vi "microfluidic_paper_controller_V1.vi"() -> ()   [LabVIEW 2016]
uses:
  <userlib>/Fluigent/Fluigent MFCS/FluigentMFCS_Full.llb/MFCS_EZ Detect.vi
  <userlib>/Fluigent/Fluigent MFCS/FluigentMFCS_Full.llb/MFCS_EZ Initialization.vi
  Gss.vi
  <vilib>/imath/engines/lvmath2/RunTimeEngine/ArithmeticOperatorToken/NIMS_ArithmeticOperator_multmx(M,CV).vi
  <instcachedir>/0/NIMS_ArithmeticOperator_multmx(M,CV)_4D43781A51B54AFABA7ECA2AD711762F.lvgen/NIMS_ArithmeticOperator_multmx(M,CV)_4D43781A51B54AFABA7ECA2AD711762F_000.vi
  <vilib>/imathl/engines/lvmath/Functions/Error Handling/Create Error.vi
  <vilib>/imath/engines/lvmath2/RunTimeEngine/IndexRead/NIMS M(R2).vi
  <instcachedir>/0/NIMS M(R2)_287818D58BD74005B29FE73CE7602B1A.lvgen/NIMS M(R2)_287818D58BD74005B29FE73CE7602B1A_000.vi
  <vilib>/imath/engines/lvmath2/RunTimeEngine/NodeEndStatement/NIMS_NodeEndStatement_Get Vector.vi
  <instcachedir>/0/NIMS_NodeEndStatement_Get Vector_6D35898B950C4E42AD3C631ACA708625.lvgen/NIMS_NodeEndStatement_Get Vector_6D35898B950C4E42AD3C631ACA708625_001.vi
  <vilib>/imath/engines/lvmath2/RunTimeEngine/NodeEndStatement/NIMS_NodeEndStatement_Output.vi
  <instcachedir>/0/NIMS_NodeEndStatement_Output_53EC0D466D134D7ABD903AC30B43404B.lvgen/NIMS_NodeEndStatement_Output_53EC0D466D134D7ABD903AC30B43404B_005.vi
  <vilib>/imath/engines/lvmath2/RunTimeEngine/ErrorHandling/NIMS_Finalize Error.vi
  <userlib>/Fluigent/Fluigent MFCS/FluigentMFCS_Full.llb/MFCS_EZ Read All Channels Pressure.vi
  <userlib>/Fluigent/Fluigent MFCS/FluigentMFCS_Full.llb/MFCS_EZ Write Channel Pressure.vi
  <userlib>/Fluigent/Fluigent MFCS/FluigentMFCS_Full.llb/MFCS_EZ Close.vi
  <vilib>/Analysis/NI_AALBase.lvlib
  <vilib>/Analysis/baseanly.llb/Mean (DBL).vi
panel:
  in  "alpha":dbl
  in  "milliseconds to wait":u32=50
  out "Set Pressure":dbl[](array[numeric])=[400.0, 400.0]
  out "Flow 1 plot 2":cluster{"[0]":dbl, "[1]":dbl}(graph)={"[0]"=400.0, "[1]"=636.4874575000703}
  out "Flow Rates":dbl[](array[numeric])=[1099.9989421021717, 636.4874575000703]
  in  "Ftot Setpoint":dbl=400.0
  in  "Vals to display":dbl=1235.0
  out "Flow 1 plot":cluster{"[0]":dbl, "[1]":dbl}(graph)={"[0]"=1099.9989421021717, "[1]"=300.0}
  out "Ferr":T1(graph)={"output[0]"=-2.2986299232843663, "output[1]"=-0.9866301071552578, "output[2]"=0.0}
  out "Pressures":dbl[](array[numeric])=[404.58697509765625, 396.3816223144531]
  in  "reset Averging":bool
  in  "Set current Pressure\n to manual pressure":bool
  out "Pressures":T2(graph)={"[0]"=404.58697509765625, "[1]"=396.3816223144531, "[2]"=400.0, "[3]"=400.0}
  in  "stop":bool=TRUE
  in  "Control Valves":enum16{"1", "2", "3", "4", "5", "6", "7", "8"}[](array[ring])=[enum."7", enum."8"]
  in  "Pressure Channels":i16[](array[numeric])=[2, 3]
  in  "Manual Pressure Set":dbl[](array[numeric])=[400.0, 400.0]
  in  "Control On":bool
  in  "F1 Setpoint":dbl=300.0
  in  "Add Ctrl?":bool
  in  "Boards":enum16{"A", "B", "C"}[](array[ring])=[enum."A", enum."A"]
  in  "Valves":enum16{"1", "2", "3", "4", "5", "6", "7", "8"}[](array[ring])=[enum."5", enum."1"]
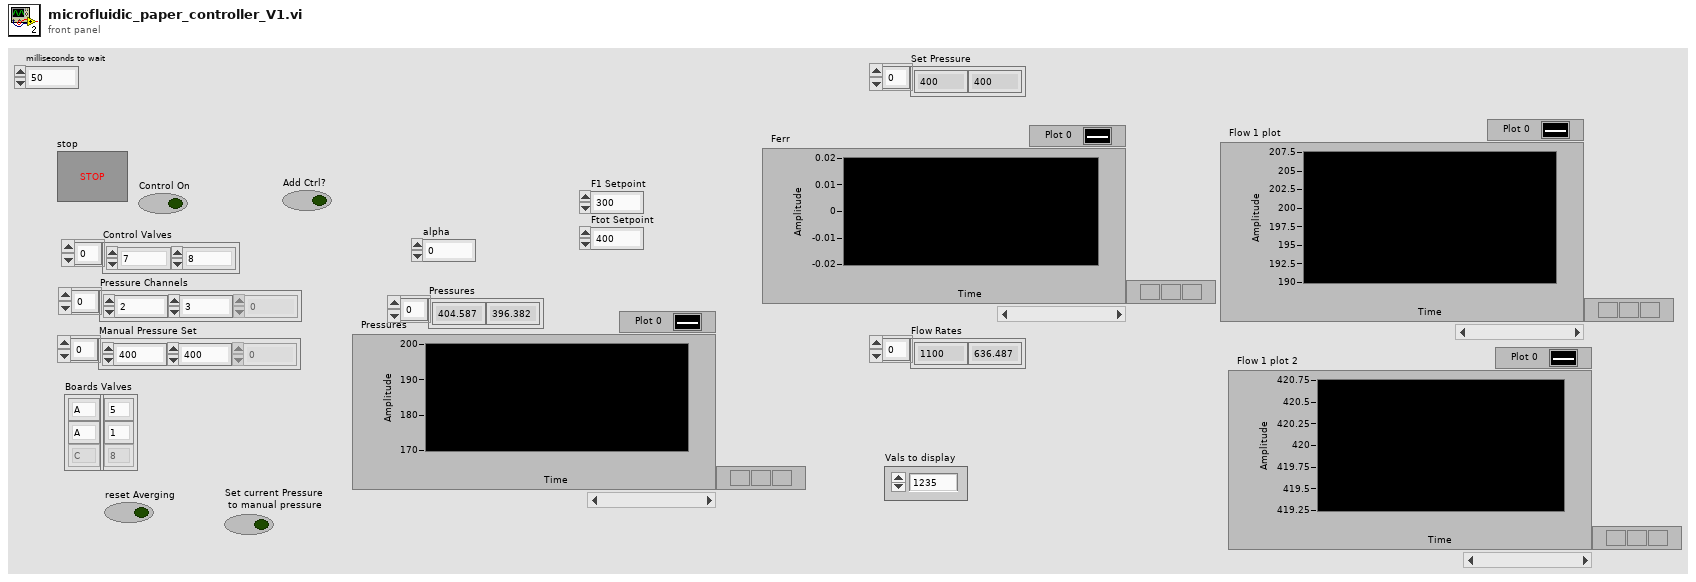
[diagram p1: front panel]
types:
  T1 = cluster{"output[0]":dbl, "output[1]":dbl, "output[2]":dbl}
  T2 = cluster{"[0]":dbl, "[1]":dbl, "[2]":dbl, "[3]":dbl}
  T3 = cluster{"relative seconds":dbl, "Pressures":dbl[], "F1 PID gains":dbl[], "FTot PID gains":dbl[], "PID On?":i16}
  T4 = typedef "_EZmfcsSN.ctl" = u16
  T5 = typedef "_EZmfcsRefNum.ctl" = refnum<k1>
  T6 = cluster{"setpoint high":dbl, "setpoint low":dbl}[]
  T7 = cluster{"err[0]":dbl, "err[1]":dbl, "err[2]":dbl}
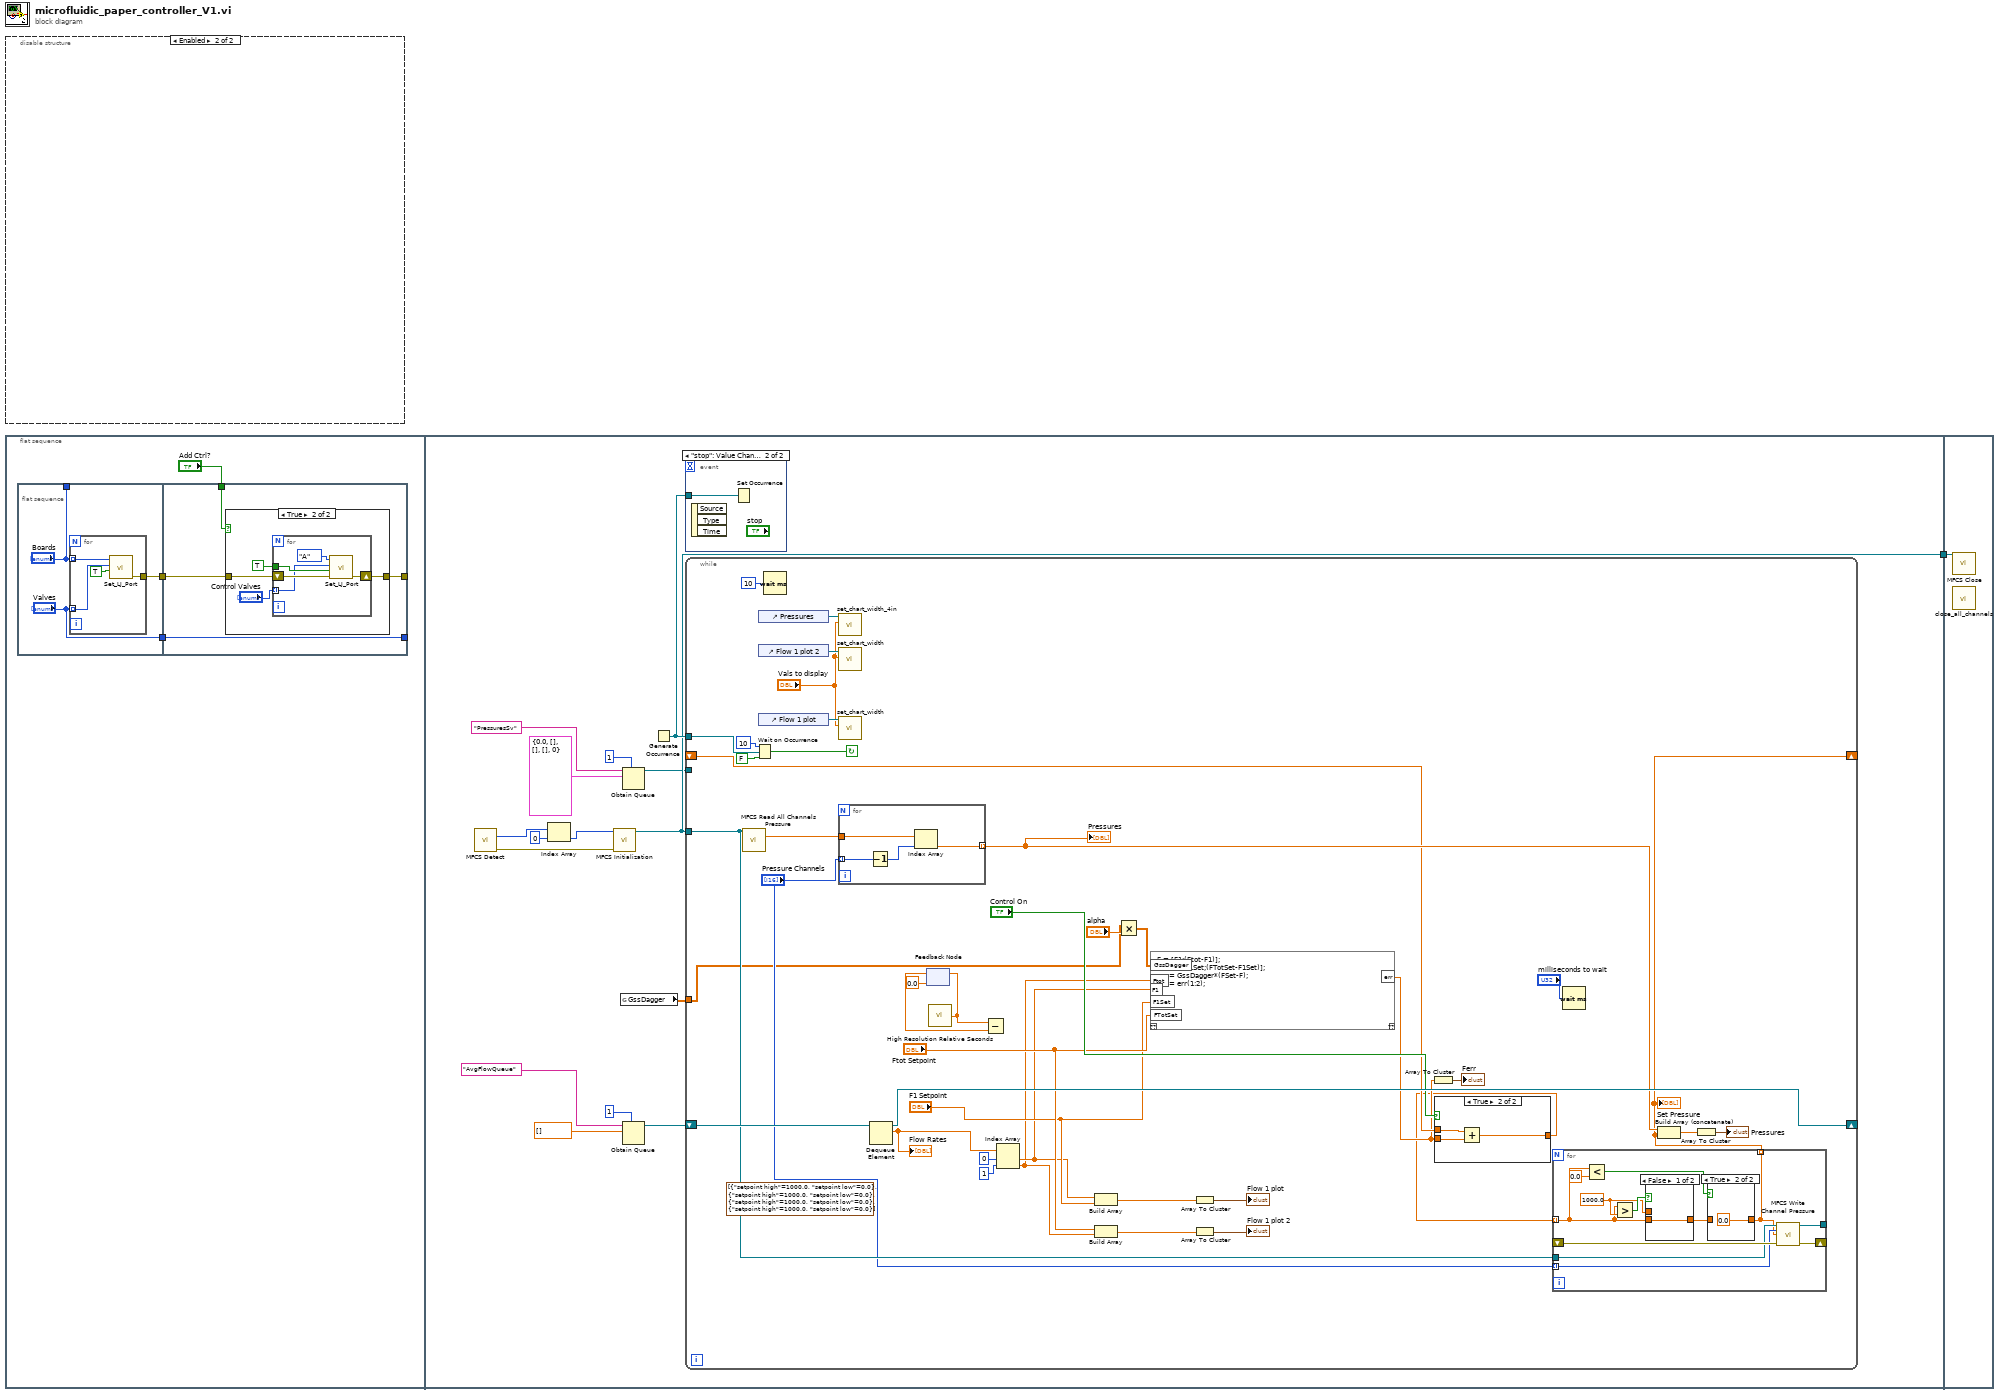
[diagram p0: block diagram]
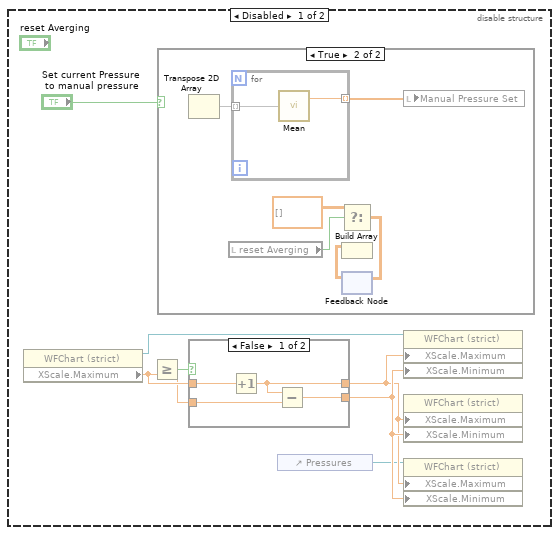
[diagram p2: hidden frame]
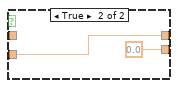
[diagram p3: hidden frame]
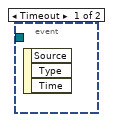
[diagram p6: hidden frame]
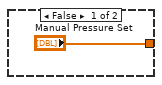
[diagram p9: hidden frame]
diagram:
  n1 = disable-structure shown="Enabled" {
    frame Disabled {
      n2 = property on="Property Node" class="WFChart (strict)"() -> (reference=w5:refnum<vi>, reference out=w6:refnum<vi>, "XScale.Maximum"=w4:dbl)  [unwired: 1 in, 1 out]
      n3 = Greater Or Equal?(y=w4) -> (x=w2:dbl, x >= y?=w3:bool)
      n4 = case shown="True" "Set current Pressure\n to manual pressure" {
        frame False {
        }
        frame True {
          n5 = Transpose 2D Array() -> (transposed array=w21:dbl[][])  [unwired: 1 in]
          n6 = local read "reset Averging"() -> (w22:bool)
          n7 = for {
            tunnel: w21 -> [w25] mode=indexing
            tunnel: [w24] -> w18 mode=indexing
            n8 = call-poly <vilib>:"Mean.vi"("X"=w25) -> ("mean"=w24:dbl)  [unwired: 1 out]
          }
          n9 = Select(t=dbl[][] [] ("appended array"), s=w22) -> (s? t:f=w19:dbl[][])  [unwired: 1 in]
          n10 = feedback-in #1(w19) -> ()
          n11 = feedback #1() -> (w23:dbl[][])  [unwired: 1 in]
          n12 = Build Array(w23) -> ()  [unwired: 1 in, 1 out]
          n13 = local write "Manual Pressure Set"(w18) -> ()
        }
      }
      n14 = case shown="False" w3 {
        tunnel: w2 -> [w13 w17]
        tunnel: w4 -> [w15 _]
        tunnel: [w12 w17] -> w9
        tunnel: [w14 0.0] -> w10
        frame False {
          n15 = Increment(x=w15) -> (x+1=w12:dbl)
          n16 = Subtract(x=w12, y=w13) -> (x-y=w14:dbl)
        }
        frame True {
        }
      }
      n17 = control-ref of="Pressures"() -> (w7:refnum<vi>)
      n18 = property on="Property Node" class="WFChart (strict)"(reference=w6, "XScale.Maximum"=w9, "XScale.Minimum"=w10) -> ()  [unwired: 1 in, 2 out]
      n19 = property on="Property Node" class="WFChart (strict)"("XScale.Maximum"=w9, "XScale.Minimum"=w10) -> (reference=w8:refnum<vi>)  [unwired: 1 in, 2 out]
      n20 = property on="Property Node" class="WFChart (strict)"(reference=w7, "XScale.Maximum"=w9, "XScale.Minimum"=w10) -> ()  [unwired: 1 in, 2 out]
    }
    frame Enabled {
    }
  }
  n21 = flat-sequence {
    tunnel: [w55] -> w1
    tunnel: w1 -> [w212]
    frame #0 {
      n22 = flat-sequence {
        tunnel: ["Boards"] -> _
        tunnel: [w31] -> w28
        tunnel: ["Valves"] -> w27
        tunnel: [w39] -> _
        tunnel: [w37] -> _
        tunnel: w28 -> [w38]
        tunnel: w27 -> [w39]
        tunnel: "Add Ctrl?" -> [w36]
        frame #0 {
          n23 = for {
            tunnel: "Valves" -> [w35] mode=indexing
            tunnel: "Boards" -> [w34] mode=indexing
            tunnel: [w32] -> w31
            n24 = call "Set_LJ_Port.vi"("State"=TRUE, "Channel"=w35, "Flowboard"=w34) -> ("error out"=w32:errorcluster)  [unwired: 8 in]
          }
        }
        frame #1 {
          n25 = case shown="True" w36 {
            tunnel: w38 -> [w40 w44]
            tunnel: [w40 w43] -> w37
            frame False {
            }
            frame True {
              n26 = for {
                tunnel: TRUE ("State") -> [w47]
                shift-right: [w48] -> w43
                shift-left: w44 -> [w49]
                tunnel: "Control Valves" -> [w46] mode=indexing
                n27 = call "Set_LJ_Port.vi"("error in"=w49, "State"=w47, "Channel"=w46, "Flowboard"=enum16{"A", "B", "C"}."A") -> ("error out"=w48:errorcluster)  [unwired: 7 in]
              }
            }
          }
        }
      }
    }
    frame #1 {
      n28 = call-poly <userlib>:"MFCS Detect.vi"() -> ("[SN MFCS_EZ]"=w64:T4[], "error out"=w62:errorcluster)  [unwired: 14 in]
      n29 = Index Array(array=w64, index=0) -> (element=w63:T4)
      n30 = call-poly <userlib>:"MFCS Initialization.vi"("SN MFCS_EZ"=w63, "error in (no error)"=w62) -> ("MFCS_EZ"=w55:T5)  [unwired: 11 in, 2 out]
      n31 = global read "Gss.vi" "GssDagger"() -> (w50:dbl[][])
      n32 = Obtain Queue(max queue size (-1, unlimited)=1, name (unnamed)="PressuresSv", element data type=T3 {"relative seconds"=0.0, "Pressures"=[], "F1 PID gains"=[], "FTot PID gains"=[], "PID On?"=0} ("output cluster")) -> (queue out=w53:refnum<queue>)  [unwired: 2 in, 2 out]
      n33 = Obtain Queue(max queue size (-1, unlimited)=1, name (unnamed)="AvgFlowQueue", element data type=dbl[] [] ("appended array")) -> (queue out=w58:refnum<queue>)  [unwired: 2 in, 2 out]
      n34 = Generate Occurrence() -> (w57:refnum<k4>)
      n35 = event shown="[1] \"stop\": Value Change" {
        selector: _ -> [_ _]
        dyn-events: _ -> [_ _]
        timeout: _ -> [_ _]
        tunnel: w57 -> [_ w65]
        event Timeout {
          n36 = event-data() -> ()  [unwired: 1 in, 3 out]
        }
        event "stop": Value Change {
          n37 = event-data() -> ()  [unwired: 1 in, 3 out]
          n38 = Set Occurrence(w65) -> ()
        }
      }
      n39 = while {
        shift-right: [w105] -> _
        shift-left: w58 -> [w106]
        tunnel: w57 -> [w100]
        tunnel: w55 -> [w97]
        shift-right: [w71] -> _
        shift-left: _ -> [w74]
        tunnel: w53 -> [_]
        tunnel: w50 -> [w67]
        stop <- w99 continue-if-true
        (unwired) T6 [{"setpoint high"=1000.0, "setpoint low"=0.0}, {"setpoint high"=1000.0, "setpoint low"=0.0}, {"setpoint high"=1000.0, "setpoint low"=0.0}, {"setpoint high"=1000.0, "setpoint low"=0.0}] ("setpoint range")
        n40 = call-poly <userlib>:"MFCS Read All Channels Pressure.vi"("MFCS_EZ"=w97) -> ("All Channels Pressure"=w95:dbl[])  [unwired: 12 in, 2 out]
        n41 = Wait on Occurrence(1:FALSE ("ignore previous (T)"), 2:w100, 3:10 ("ms timeout (-1)")) -> (0:w99:bool)
        n42 = control-ref of="Pressures"() -> (w94:refnum<vi>)
        n43 = control-ref of="Flow 1 plot 2"() -> (w81:refnum<vi>)
        n44 = control-ref of="Flow 1 plot"() -> (w80:refnum<vi>)
        n45 = Wait (ms)(milliseconds to wait=u32 10) -> ()  [unwired: 1 out]
        n46 = call "set_chart_width_4in.vi"("Values to Display"="Vals to display", "Ref In"=w94) -> ()  [unwired: 10 in]
        n47 = call "set_chart_width.vi"("Values to Display"="Vals to display", "Ref In"=w81) -> ()  [unwired: 10 in]
        n48 = call "set_chart_width.vi"("Values to Display"="Vals to display", "Ref In"=w80) -> ()  [unwired: 10 in]
        n49 = for {
          tunnel: "Pressure Channels" -> [w190] mode=indexing
          tunnel: w95 -> [w191]
          tunnel: [w188] -> w83 mode=indexing
          n50 = Decrement(x=w190) -> (x-1=w189:i16)
          n51 = Index Array(array=w191, index=w189) -> (element=w188:dbl)
        }
        "Pressures" <- w83
        n52 = Dequeue Element(queue=w106) -> (queue out=w105:refnum<queue>, element=w90:dbl[])  [unwired: 2 in, 2 out]
        "Flow Rates" <- w90
        n53 = feedback #2(0.0 ("relative seconds")) -> (w103:dbl)
        n54 = call <vilib>:"High Resolution Relative Seconds.vi"() -> ("relative seconds"=w85:dbl)
        n55 = feedback-in #2(w85) -> ()
        n56 = Subtract(x=w85, y=w103) -> ()  [unwired: 1 out]
        n57 = Index Array(array=w90, index #1=0 ("index"), index #2=1 ("index")) -> (element #1=w76:dbl, element #2=w75:dbl)
        n58 = Build Array(w76, "F1 Setpoint") -> (w89:dbl[])
        n59 = Build Array("Ftot Setpoint", w75) -> (w87:dbl[])
        n60 = Multiply(x=w67, y="alpha") -> (x*y=w66:dbl[][])
        n61 = mathscript code="F = [F1;(Ftot-F1)];\nFSet = [F1Set;(FTotSet-F1Set)];\nerr = GssDagger*(FSet-F);\nerr = err(1:2);"("GssDagger"=w66, "Ftot"=w75, "F1"=w76, "F1Set"="F1 Setpoint", "FTotSet"="Ftot Setpoint") -> ("err"=w73:dbl[])  [unwired: 1 in, 1 out]
        n62 = Array To Cluster(array=w89) -> (cluster=→"Flow 1 plot":cluster{"[0]":dbl, "[1]":dbl})
        n63 = Array To Cluster(array=w87) -> (cluster=→"Flow 1 plot 2":cluster{"[0]":dbl, "[1]":dbl})
        n64 = Array To Cluster(array=w73) -> (cluster=→"Ferr":T7)
        n65 = case shown="True" "Control On" {
          tunnel: w73 -> [_ w209]
          tunnel: w74 -> [_ w211]
          tunnel: ["Manual Pressure Set" w210] -> w72
          frame False {
          }
          frame True {
            n66 = Add(x=w211, y=w209) -> (x+y=w210:dbl[])
          }
        }
        n67 = for {
          shift-right: [w202] -> _
          shift-left: _ -> [w203]
          tunnel: [w201] -> _
          tunnel: "Pressure Channels" -> [w200] mode=indexing
          tunnel: w72 -> [w195] mode=indexing
          tunnel: w97 -> [w199]
          tunnel: [w192] -> w71 mode=indexing
          w197 = 1000.0 ("y")
          n68 = Less?(x=w195, y=0.0) -> (x < y?=w194:bool)
          n69 = Greater?(x=w195, y=w197) -> (0:w198:bool)
          n70 = case shown="False" w198 {
            tunnel: w195 -> [w206 _]
            tunnel: [w206 w207] -> w193
            tunnel: w197 -> [_ w207]
            frame False {
            }
            frame True {
            }
          }
          n71 = case shown="True" w194 {
            tunnel: w193 -> [w204 _]
            tunnel: [w204 0.0 ("y")] -> w192
            frame False {
            }
            frame True {
            }
          }
          n72 = call-poly <userlib>:"MFCS Write Channel Pressure.vi"("MFCS_EZ"=w199, "Channel Number (default=1)"=w200, "Pressure (mBar)"=w192, "error in (no error)"=w203) -> ("MFCS_EZ out"=w201:T5, "error out"=w202:errorcluster)  [unwired: 10 in]
        }
        "Set Pressure" <- w71
        n73 = Wait (ms)(milliseconds to wait="milliseconds to wait") -> ()  [unwired: 1 out]
        n74 = Build Array (concatenate)(w83, w71) -> (w82:dbl[])
        n75 = Array To Cluster(array=w82) -> (cluster=→"Pressures":T2)
      }
    }
    frame #2 {
      n76 = call-poly <userlib>:"MFCS Close.vi"("MFCS_EZ"=w212) -> ()  [unwired: 14 in, 1 out]
      n77 = call "close_all_channels.vi"() -> ()  [unwired: 12 in]
    }
  }
